vi "SetFltrMode.vi"(8 "错误输入（无错误）":errorcluster, 10 "滤波模式索引值":u16) -> (0 "错误输出":errorcluster)   [LabVIEW 2014]
uses:
  X86Dll/ZXUTConfigMgr.dll
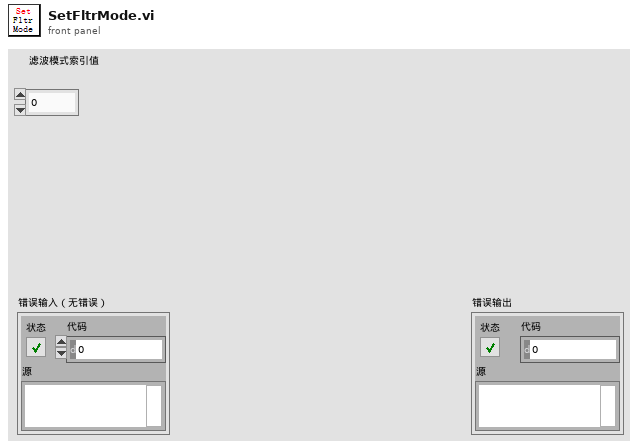
[diagram p1: front panel]
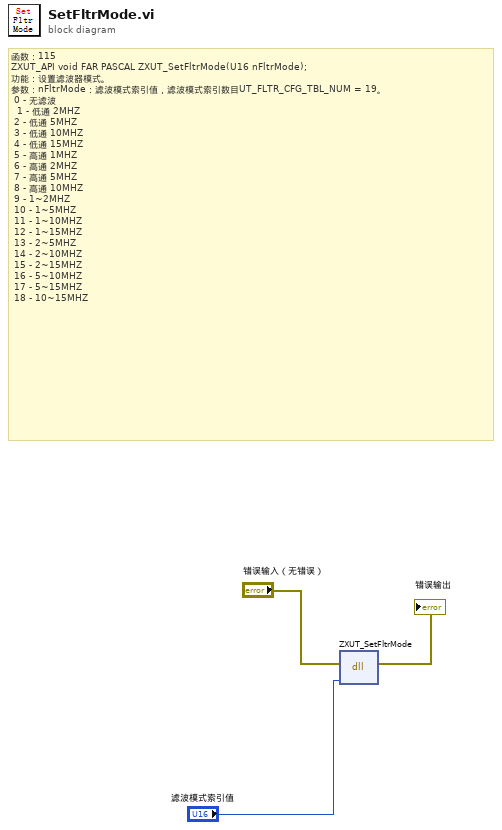
[diagram p0: block diagram]
diagram:
  # "函数：115\nZXUT_API void\tFAR PASCAL ZXUT_SetFltrMode(U16 nFltrMode);\n功能：设置滤波器模式。\n参数：nFltrMode：滤波模式索引值，滤波模式索引数目UT_FLTR_CFG_TBL_NUM = 19。\n\t0 - 无滤波\n \t1 - 低通 2MHZ\n\t2 - 低通 5MHZ\n\t3 - 低通 10MHZ\n\t4 - 低通 15MHZ\n\t5 - 高通 1MHZ\n\t6 - 高通 2MHZ\n\t7 - 高通 5MHZ\n\t8 - 高通 10MHZ\n\t9 - 1~2MHZ\n\t10 - 1~5MHZ\n\t11 - 1~10MHZ\n\t12 - 1~15MHZ\n\t13 - 2~5MHZ\n\t14 - 2~10MHZ\n\t15 - 2~15MHZ\n\t16 - 5~10MHZ\n\t17 - 5~15MHZ\n\t18 - 10~15MHZ"
  n1 = dll-call lib="D:/Software/Utrasonic on-line monitoring/X86Dll/ZXUTConfigMgr.dll" fn="ZXUT_SetFltrMode"(error in="错误输入（无错误）", "nFltrMode"="滤波模式索引值") -> (error out=→"错误输出":errorcluster)  [unwired: 4 in, 1 out]
